vi "Write Jump To.vi"(8 "error in (no error)":errorcluster, 10 "Jump To":i32, 11 "Conditional Jump Step in":refnum<class "Conditional Jump Step.lvclass">) -> (0 "error out":errorcluster, 3 "Conditional Jump Step out":refnum<class "Conditional Jump Step.lvclass">)   [LabVIEW 2015, in "Conditional Jump Step.lvclass"]
uses:
  Conditional Jump Step.lvclass
  Conditional Jump Step.lvclass/Conditional Jump Step.ctl
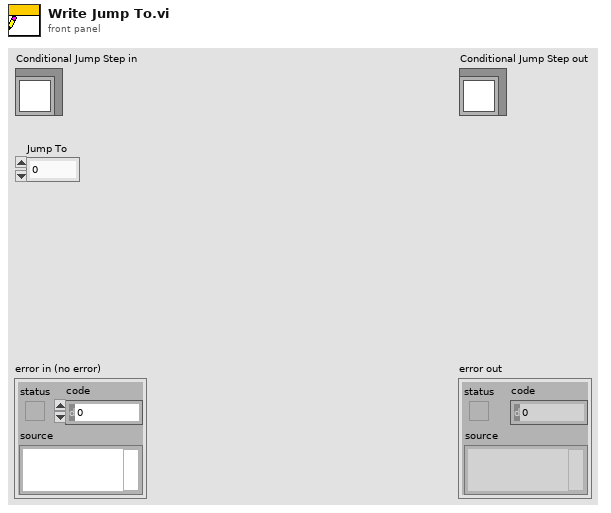
[diagram p1: front panel]
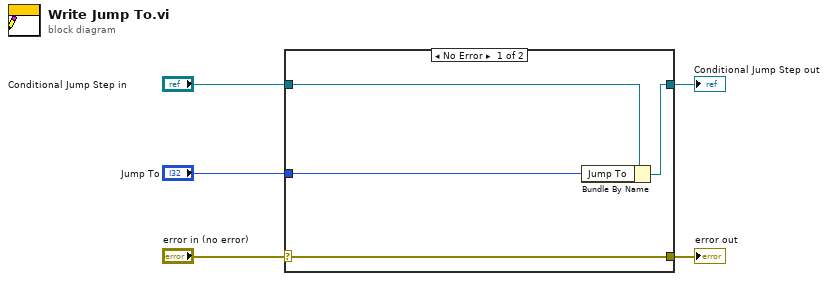
[diagram p0: block diagram]
diagram:
  n1 = case shown="No Error" "error in (no error)" {
    selector: "error in (no error)" -> [w9 w10]
    tunnel: [w9 w10] -> w4
    tunnel: [w7 w11] -> w2
    tunnel: "Conditional Jump Step in" -> [w8 w11]
    tunnel: "Jump To" -> [w6 _]
    frame No Error {
      n2 = Bundle By Name(cluster=w8, "Jump To"=w6) -> (w7:refnum<class "Conditional Jump Step.lvclass">)
    }
    frame Error {
    }
  }
  "error out" <- w4
  "Conditional Jump Step out" <- w2
